vi "Avantes - AVS_GetLambda.vi"(8 "error in (no error)":errorcluster, 11 "AVS Settings In":T1) -> (0 "error out":errorcluster, 2 "a_pWaveLength":dbl[](array[numeric]), 3 "AVS Settings Out":T1)   [LabVIEW 2013, in "Avantes Spectrometer Functions.lvlib"]
uses:
  Avantes Spectrometer Functions.lvlib
  AVS settings.ctl
  IRRAD-DLL/AVSirrad.lvlib
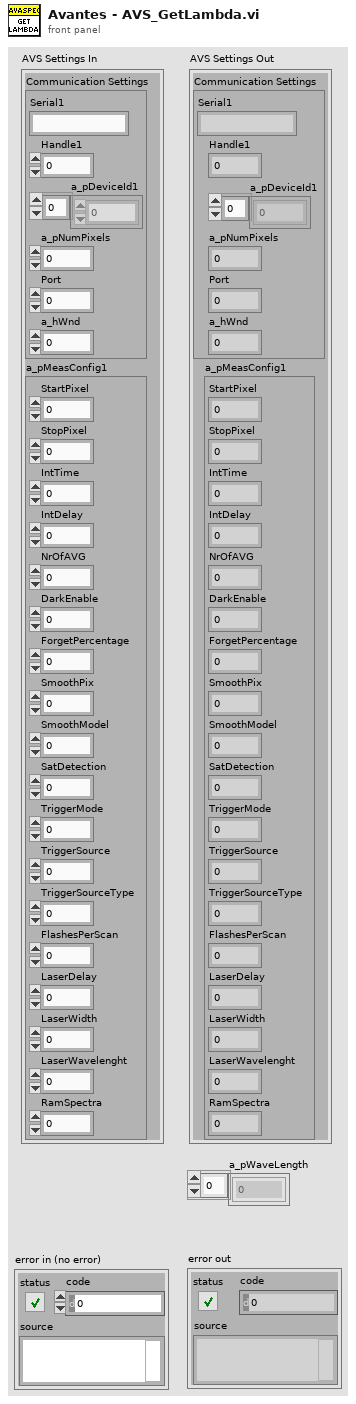
[diagram p1: front panel]
types:
  T1 = typedef "AVSirrad.lvlib/AVS settings.ctl" = cluster{"Communication Settings":cluster{"Serial1":string, "Handle1":i32, "a_pDeviceId1":u8[], "a_pNumPixels":u16, "Port":i32, "a_hWnd":i32}, "a_pMeasConfig1":cluster{"StartPixel":u16, "StopPixel":u16, "IntTime":sgl, "IntDelay":u32, "NrOfAVG":u32, "DarkEnable":u8, "ForgetPercentage":u8, "SmoothPix":u16, "SmoothModel":u8, "SatDetection":u8, "TriggerMode":u8, "TriggerSource":u8, "TriggerSourceType":u8, "FlashesPerScan":u16, "LaserDelay":u32, "LaserWidth":u32, "LaserWavelenght":sgl, "RamSpectra":u16}}
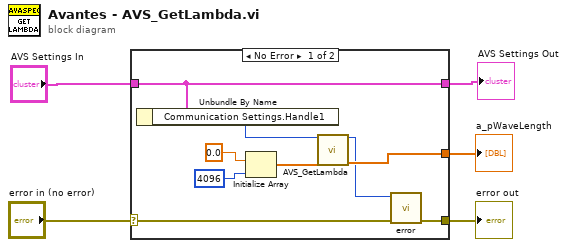
[diagram p0: block diagram]
diagram:
  n1 = case shown="No Error" "error in (no error)" {
    selector: "error in (no error)" -> [w8 w16]
    tunnel: [w11 w15] -> w1
    tunnel: "AVS Settings In" -> [w11 w15]
    tunnel: [w7 w16] -> w4
    tunnel: [w9 _] -> w3
    frame No Error {
      n2 = Unbundle By Name(w11) -> ("Communication Settings.Handle1"=w10:i32)
      n3 = Initialize Array(0.0 ("element"), 4096 ("dimension size")) -> (w12:dbl[])
      n4 = call "AVS_GetLambda.vi"("a_hDevice"=w10, "a_pWaveLength"=w12) -> ("Output Value"=w6:i32, "a_pWaveLength"=w9:dbl[])  [unwired: 12 in]
      n5 = call "error.vi"("error in (no error)"=w8, "Output Value"=w6) -> ("error out"=w7:errorcluster)  [unwired: 9 in]
    }
    frame Error {
    }
  }
  "error out" <- w4
  "a_pWaveLength" <- w3
  "AVS Settings Out" <- w1
